vi "getHeater.vi"(6 "Channel":i32, 8 "error in (no error)":errorcluster, 11 "Instrument.Cryostat in":refnum<class "Instrument.Cryostat.lvclass">) -> (0 "error out":errorcluster, 1 "Status":string, 2 "Current (A)":dbl, 3 "Instrument.Cryostat out":refnum<class "Instrument.Cryostat.lvclass">)   [LabVIEW 2019, in "Instrument.Cryostat.lvclass"]
uses:
  Instrument.Cryostat.lvclass
  Instrument/Instrument.lvclass
  Typedefs/getHeater--cluster.ctl
  cea45727-4822-453d-9f84-850d5cfe7c38.vi
  C:/Users/patrick/Documents/GitHub/Instrument-Framework/lvsrc/Instrument/Instrument.lvclass
  C:/Program Files (x86)/National Instruments/LabVIEW 2019/vi.lib/JKI/JKI SMO/SMO/SMO.lvclass
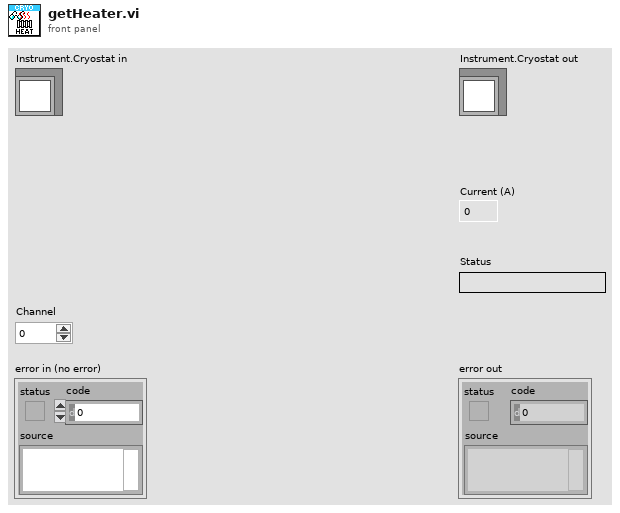
[diagram p1: front panel]
types:
  T1 = typedef "Instrument.Cryostat.lvclass/getHeater--cluster.ctl" = cluster{"current":dbl, "status":string}
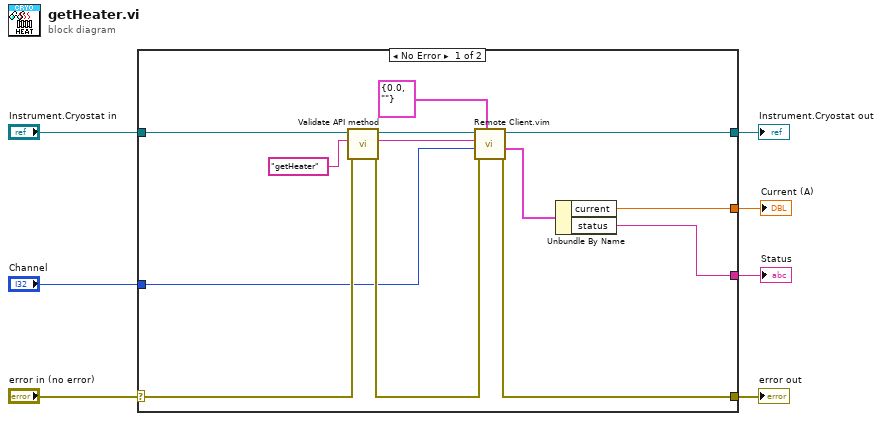
[diagram p0: block diagram]
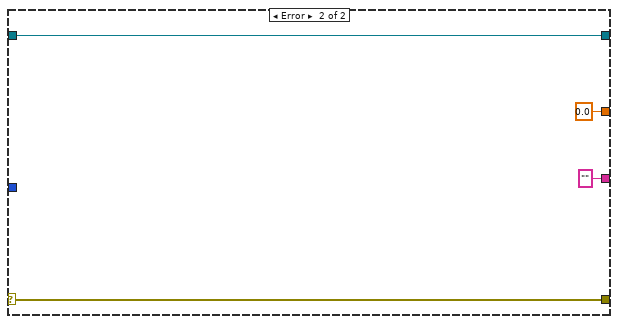
[diagram p2: hidden frame]
diagram:
  n1 = case shown="No Error" "error in (no error)" {
    selector: "error in (no error)" -> [w14 w24]
    tunnel: [w9 w24] -> w6
    tunnel: [w15 w23] -> w4
    tunnel: "Instrument.Cryostat in" -> [w16 w23]
    tunnel: [w13 0.0 ("Current")] -> w3
    tunnel: [w12 "" ("Status")] -> w2
    tunnel: "Channel" -> [w10 _]
    frame No Error {
      n2 = call "Validate API method.vi"("error in (no error)"=w14, "Command in"="getHeater" ("error message (\"\")"), "Instrument in"=w16) -> ("error out"=w11:errorcluster, "command out"=w19:string, "Instrument out"=w18:refnum<class "Instrument.Cryostat.lvclass">)  [unwired: 6 in]
      n3 = call "Remote Client.vim"("Command out"=w19, "Data Out type"=T1 {"current"=0.0, "status"=""} ("getHeat"), "error in (no error)"=w11, "Data in"=w10, "Instrument in"=w18) -> ("error out"=w9:errorcluster, "Data out"=w17:T1, "Instrument out"=w15:refnum<class "Instrument.Cryostat.lvclass">)  [unwired: 4 in]
      n4 = Unbundle By Name(w17) -> ("current"=w13:dbl, "status"=w12:string)
    }
    frame Error {
    }
  }
  "error out" <- w6
  "Instrument.Cryostat out" <- w4
  "Current (A)" <- w3
  "Status" <- w2
